vi "Digital output.vi"(7 "Boolean":bool, 8 "error in":errorcluster, 9 "milliseconds to wait":u32, 10 "data":u32[](array[numeric]), 11 "task/channels in":refnum<k21>) -> (0 "error out":errorcluster)   [LabVIEW 2013]
uses:
  <vilib>/DAQmx/write.llb/DAQmx Write (Digital 1D U32 NChan 1Samp).vi
  <vilib>/DAQmx/miscellaneous.llb/DAQmx Fill In Error Info.vi
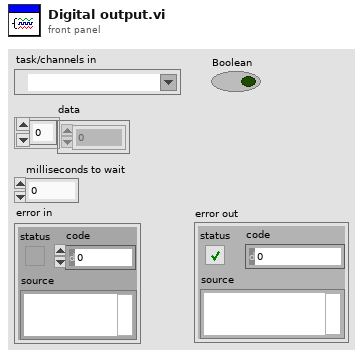
[diagram p1: front panel]
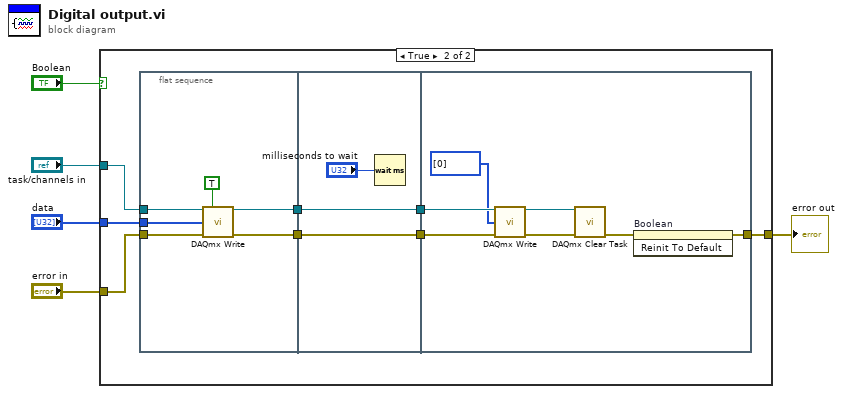
[diagram p0: block diagram]
diagram:
  n1 = case shown="True" "Boolean" {
    tunnel: [w6 w10] -> w1
    tunnel: "data" -> [_ w9]
    tunnel: "task/channels in" -> [_ w8]
    tunnel: "error in" -> [w6 w7]
    frame False {
    }
    frame True {
      n2 = flat-sequence {
        tunnel: w9 -> [w20]
        tunnel: [w18] -> w14
        tunnel: [w17] -> w13
        tunnel: w8 -> [w16]
        tunnel: w7 -> [w15]
        tunnel: w14 -> [w23]
        tunnel: w13 -> [w22]
        tunnel: [w23] -> w12
        tunnel: [w22] -> w11
        tunnel: w12 -> [w30]
        tunnel: w11 -> [w29]
        tunnel: [w24] -> w10
        frame #0 {
          n3 = call-poly <vilib>:"DAQmx Write.vi"("task/channels in"=w16, "auto start"=TRUE, "data"=w20, "error in"=w15) -> ("task out"=w18:refnum<k21>, "error out"=w17:errorcluster)  [unwired: 9 in, 1 out]
        }
        frame #1 {
          n4 = Wait (ms)(milliseconds to wait="milliseconds to wait") -> ()  [unwired: 1 out]
        }
        frame #2 {
          n5 = call-poly <vilib>:"DAQmx Write.vi"("task/channels in"=w30, "data"=u32[] [0], "error in"=w29) -> ("task out"=w27:refnum<k21>, "error out"=w26:errorcluster)  [unwired: 10 in, 1 out]
          n6 = call <vilib>:"DAQmx Clear Task.vi"("task in"=w27, "error in"=w26) -> ("error out"=w25:errorcluster)  [unwired: 13 in]
          n7 = invoke on="Boolean" class="Bool (strict)" method="Reinit To Default"(error in=w25) -> (error out=w24:errorcluster)  [unwired: 2 in, 2 out]
        }
      }
    }
  }
  "error out" <- w1
